vi "Prober_InitialiseUI.vi"(8 "error in (no error)":errorcluster, 11 "VeloxTeslaProbestation in":refnum<class "VeloxTeslaProbestation.lvclass">) -> (0 "error out":errorcluster, 3 "VeloxTeslaProbestation out":refnum<class "VeloxTeslaProbestation.lvclass">)   [LabVIEW 2018, in "VeloxTeslaProbestation.lvclass"]
uses:
  VeloxTeslaProbestation.lvclass
  VeloxTeslaProbestation.lvclass/VeloxTeslaProbestation.ctl
  Desktop/Kvasnicka/test_labview_library/Integration_toolkit_library/CascadeProbestation.lvlib
panel:
  out "Connected device (ResourceName)":string
  in  "Stop Button":bool
  in  "Needles Clear":bool
  in  "Nucleus":bool
  # "Starting Probe Station Control Interface"
  # "This step will register the labview application to the VELOX software. If the labview was not exitted properly with (proper close of communitation), it will fail and disconnect properly. Next time it should work."
  # "Before continuing, please confirm the following:"
  # "1. Velox is running on the probestation PC"
  # "2. No device on chuck and needles are clear"
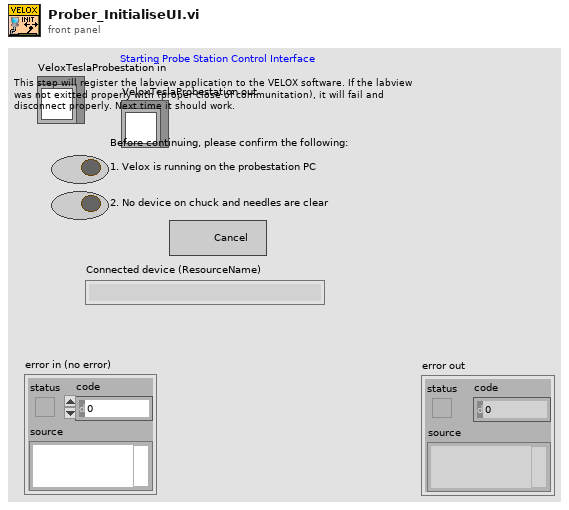
[diagram p1: front panel]
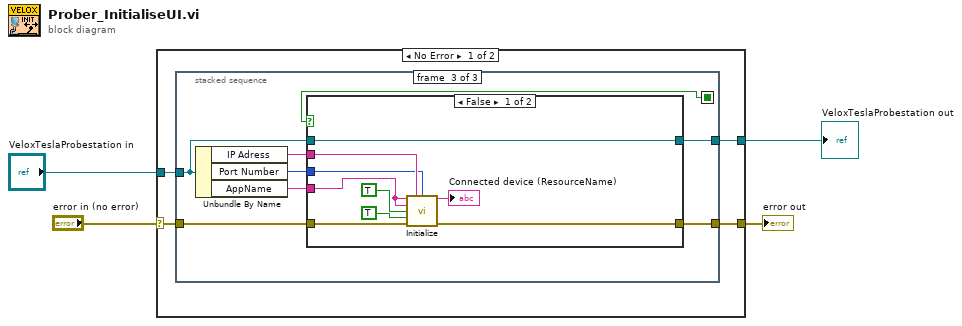
[diagram p0: block diagram]
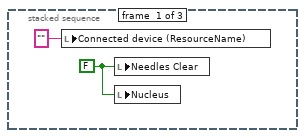
[diagram p2: hidden frame]
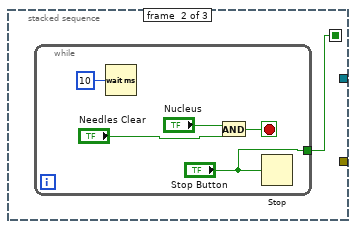
[diagram p3: hidden frame]
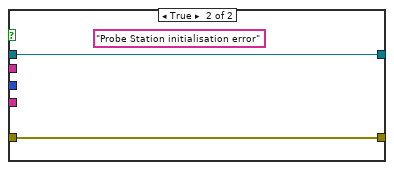
[diagram p4: hidden frame]
diagram:
  n1 = case shown="No Error" "error in (no error)" {
    selector: "error in (no error)" -> [w8 w37]
    tunnel: [w7 w37] -> w2
    tunnel: [w6 w36] -> w4
    tunnel: "VeloxTeslaProbestation in" -> [w5 w36]
    frame No Error {
      n2 = stacked-sequence {
        seq-local: [_ w11 _] -> [_ _ w24]
        tunnel: w8 -> [_ _ w17]
        tunnel: [_ _ w23] -> w7
        tunnel: [_ _ w22] -> w6
        tunnel: w5 -> [_ _ w18]
        frame #0 {
          w10 = FALSE
          n3 = local write "Connected device (ResourceName)"("" ("Connected device (ResourceName)")) -> ()
          n4 = local write "Needles Clear"(w10) -> ()
          n5 = local write "Nucleus"(w10) -> ()
        }
        frame #1 {
          n6 = while {
            tunnel: ["Stop Button"] -> w11
            stop <- w16 stop-if-true
            n7 = Wait (ms)(milliseconds to wait=u32 10) -> ()  [unwired: 1 out]
            n8 = And(x="Nucleus", y="Needles Clear") -> (x .and. y?=w16:bool)
            n9 = Stop(stop? (T)="Stop Button") -> ()
          }
        }
        frame #2 {
          n10 = Unbundle By Name(w18) -> ("IP Adress"=w21:string, "Port Number"=w20:i32, "AppName"=w19:string)
          n11 = case shown="False" w24 {
            tunnel: w17 -> [w31 w34]
            tunnel: [w30 w34] -> w23
            tunnel: [w33 w35] -> w22
            tunnel: w18 -> [w33 w35]
            tunnel: w21 -> [w28 _]
            tunnel: w20 -> [w27 _]
            tunnel: w19 -> [w26 _]
            frame False {
              n12 = call "Initialize.vi"("AppName"=w26, "IP Adress"=w28, "Port Number"=w27, "GroupName"=w26, "EnableNotification"=TRUE, "Use Socket Connection"=TRUE, "Error In (no error)"=w31) -> ("ResourceName"=→"Connected device (ResourceName)":string, "Error Out"=w30:errorcluster)  [unwired: 7 in]
            }
            frame True {
              (unwired) "Probe Station initialisation error" ("Error String IN")
            }
          }
        }
      }
    }
    frame Error {
    }
  }
  "error out" <- w2
  "VeloxTeslaProbestation out" <- w4
